vi "Get Terminal Mode Strings Values.vi"(11 "Terminal Mode Display Values":T1[](array[typedef])) -> (3 "Terminal Mode RSI Values":u32[](array[numeric]))   [LabVIEW 2017, in "Modules.lvlib" / "9209.lvclass"]
uses:
  9209.lvclass
  Terminal mode.ctl
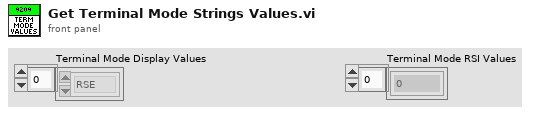
[diagram p1: front panel]
types:
  T1 = typedef "Modules.lvlib/9209.lvclass/Terminal mode.ctl" = enum16{"RSE", "DIFF"}
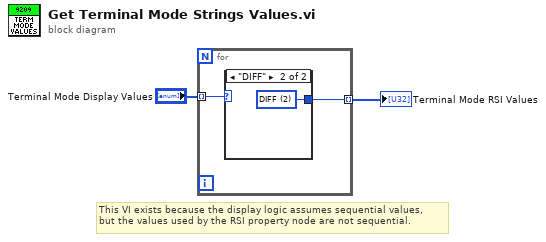
[diagram p0: block diagram]
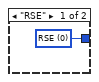
[diagram p2: hidden frame]
diagram:
  # "This VI exists because the display logic assumes sequential values, \nbut the values used by the RSI property node are not sequential."
  n1 = for {
    tunnel: "Terminal Mode Display Values" -> [w4] mode=indexing
    tunnel: [w3] -> w1 mode=indexing
    n2 = case shown="\"DIFF\"" w4 {
      tunnel: [w5 w6] -> w3
      frame "RSE" {
        w5 = u32 0 items=["RSE"=0, "DIFF"=2] ("AI0:Terminal mode")
      }
      frame "DIFF" {
        w6 = u32 2 items=["RSE"=0, "DIFF"=2] ("AI0:Terminal mode")
      }
    }
  }
  "Terminal Mode RSI Values" <- w1
